vi "GridParam(SubVI).vi"(10 "Numeric in":i32, 11 "ItemNames":string[][](array[string])) -> (1 "Img Current":dbl, 2 "Bias":dbl, 3 "GridSettings":T1)   [LabVIEW 2014]
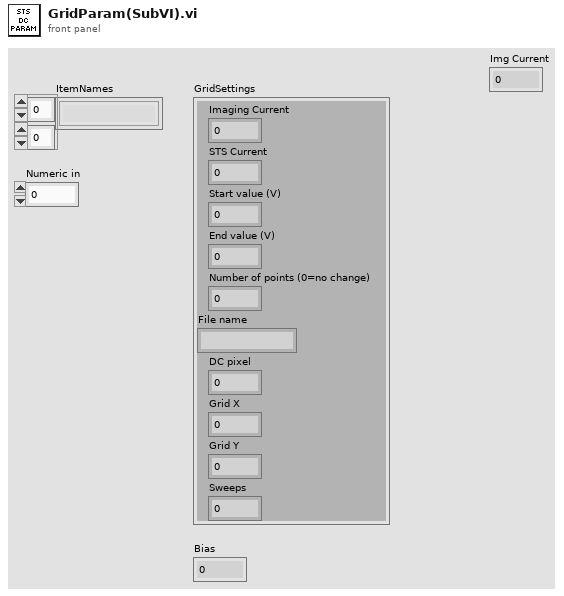
[diagram p1: front panel]
types:
  T1 = cluster{"Imaging Current":sgl, "STS Current":sgl, "Start value (V)":sgl, "End value (V)":sgl, "Number of points (0=no change)":i32, "File name":string, "DC pixel":dbl, "Grid X":dbl, "Grid Y":dbl, "Sweeps":dbl}
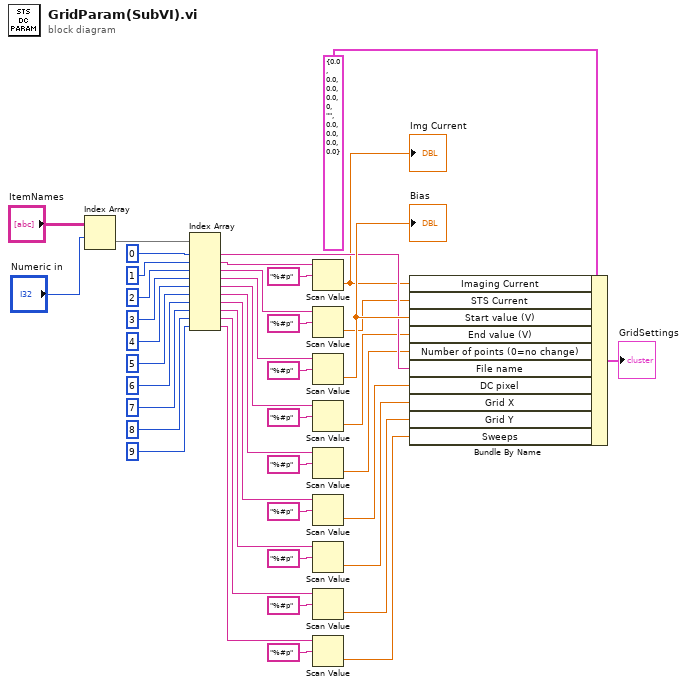
[diagram p0: block diagram]
diagram:
  n1 = Index Array(array="ItemNames", index (row)="Numeric in") -> (element=w8:string[])  [unwired: 1 in]
  n2 = Index Array(array=w8, index #1=0 ("index"), index #2=1 ("index"), index #3=2 ("index"), index #4=3 ("index"), index #5=4 ("index"), index #6=5 ("index"), index #7=6 ("index"), index #8=7 ("index"), index #9=8 ("index"), index #10=9 ("index")) -> (element #1=w36:string, element #2=w18:string, element #3=w20:string, element #4=w22:string, element #5=w23:string, element #6=w24:string, element #7=w25:string, element #8=w28:string, element #9=w29:string, element #10=w39:string)
  n3 = Scan Value(string=w18, format string="%#p") -> (value=w19:dbl)  [unwired: 1 in, 1 out]
  "Img Current" <- w19
  n4 = Scan Value(string=w20, format string="%#p") -> (value=w21:dbl)  [unwired: 1 in, 1 out]
  n5 = Scan Value(string=w22, format string="%#p") -> (value=w42:dbl)  [unwired: 1 in, 1 out]
  "Bias" <- w42
  n6 = Scan Value(string=w23, format string="%#p") -> (value=w32:dbl)  [unwired: 1 in, 1 out]
  n7 = Scan Value(string=w24, format string="%#p") -> (value=w33:dbl)  [unwired: 1 in, 1 out]
  n8 = Scan Value(string=w25, format string="%#p") -> (value=w34:dbl)  [unwired: 1 in, 1 out]
  n9 = Scan Value(string=w28, format string="%#p") -> (value=w31:dbl)  [unwired: 1 in, 1 out]
  n10 = Scan Value(string=w29, format string="%#p") -> (value=w30:dbl)  [unwired: 1 in, 1 out]
  n11 = Scan Value(string=w39, format string="%#p") -> (value=w40:dbl)  [unwired: 1 in, 1 out]
  n12 = Bundle By Name(cluster=T1 {"Imaging Current"=0.0, "STS Current"=0.0, "Start value (V)"=0.0, "End value (V)"=0.0, "Number of points (0=no change)"=0, "File name"="", "DC pixel"=0.0, "Grid X"=0.0, "Grid Y"=0.0, "Sweeps"=0.0} ("GridSettings"), "Imaging Current"=w19, "STS Current"=w21, "Start value (V)"=w42, "End value (V)"=w32, "Number of points (0=no change)"=w33, "File name"=w36, "DC pixel"=w34, "Grid X"=w31, "Grid Y"=w30, "Sweeps"=w40) -> (→"GridSettings":T1)
